vi "PIV_Stats_Single_Fast.vi"(0 "Data Folder":path=path "T:/Ensight_Data/NACA0015/NACA0015_NM_B/Test_A", 1 "PIV Meas Plane":enum16{"XY", "YZ", "XZ"}(ring)=enum."XZ", 2 "Row number":i32=1, 5 "Output Directory":path=path "T:/Ensight_Data/NACA0015/NACA0015_NM_B", 7 "XYZ Translation":dbl[](array[numeric])=[200.0, 8.0, -30.0], 9 "Case Name":string="Test_A_Case", 11 "PIV Freq (Hz)":dbl=7.25, 12 "Invert U":bool=TRUE, 13 "Invert V":bool) -> (4 "Progress Bar":i32(slide) scale=0.0..100.0, 6 "Status":string, 10 "# total vectors":i32=9858)   [LabVIEW 2022 SP3]
uses:
  <vilib>/Utility/error.llb/DialogType.ctl
  <vilib>/Analysis/1siggen.llb/Ramp Pattern by Samples.vi
  <vilib>/Utility/error.llb/Trim Whitespace One-Sided.vi
  <vilib>/Analysis/NI_AALBase.lvlib
panel:
  out "Data Array (spot,Var)":dbl[][](array[numeric])
  out "File Paths":path[](array[path])
  out "Position Array (XYZ,spot)":dbl[][](array[numeric])
  out "Variable Names":string[](array[string])=["Record_Length", "CHC", "u_ms", "v_ms", "time_s", "Vel_mag_ms", "Turb_Stats_U_ms", "Turb_Stats_u2_m2s2", "Turb_Stats_u3_m3s3", "Turb_Stats_u4_m4s4", "Turb_Stats_TurbU_%", "Turb_Stats_Skew_u", "Turb_Stats_Kurt_u", "Turb_Stats_V_ms", "Turb_Stats_v2_m2s2", "Turb_Stats_v3_m3s3", "Turb_Stats_v4_m4s4", "Turb_Stats_TurbV_%", "Turb_Stats_Skew_v", "Turb_Stats_Kurt_v", "Turb_Stats_u2v2_m4s4", "Turb_Stats_uv3_m4s4", "Turb_Stats_u3v_m4s4", "Turb_Stats_uv2_m3s3", "Turb_Stats_u2v_m3s3", "Turb_Stats_uv_cc", "Turb_Stats_uv", "Turb_Stats_TKE_J", "Turb_Stats_Error_U_ms", "Turb_Stats_Error_u2_m2s2", "Turb_Stats_Error_u3_m3s3", "Turb_Stats_Error_u4_m4s4", "Turb_Stats_Error_TurbU_%", "Turb_Stats_Error_Skew_u", "Turb_Stats_Error_Kurt_u", "Turb_Stats_Error_V_ms", "Turb_Stats_Error_v2_m2s2", "Turb_Stats_Error_v3_m3s3", "Turb_Stats_Error_v4_m4s4", "Turb_Stats_Error_TurbV_%", "Turb_Stats_Error_Skew_v", "Turb_Stats_Error_Kurt_v", "Turb_Stats_Error_u2v2_m4s4", "Turb_Stats_Error_uv3_m4s4", "Turb_Stats_Error_u3v_m4s4", "Turb_Stats_Error_uv2_m3s3", "Turb_Stats_Error_u2v_m3s3", "Turb_Stats_Error_uv_cc", "Turb_Stats_Error_uv", "Turb_Stats_Error_TKE_J"]
  out "time s":dbl[](array[numeric])=[0.0, 0.20689655172413793, 0.41379310344827586]
  out "File Array":path[](array[path])=[path "T:/Ensight_Data/NACA0015/NACA0015_NM_A/Test_A_Trans/New folder/Test_A000000.T076.D000.P000.H000.L.vec", path "T:/Ensight_Data/NACA0015/NACA0015_NM_A/Test_A_Trans/New folder/Test_A000001.T076.D000.P000.H000.L.vec", path "T:/Ensight_Data/NACA0015/NACA0015_NM_A/Test_A_Trans/New folder/Test_A000002.T076.D000.P000.H000.L.vec"]
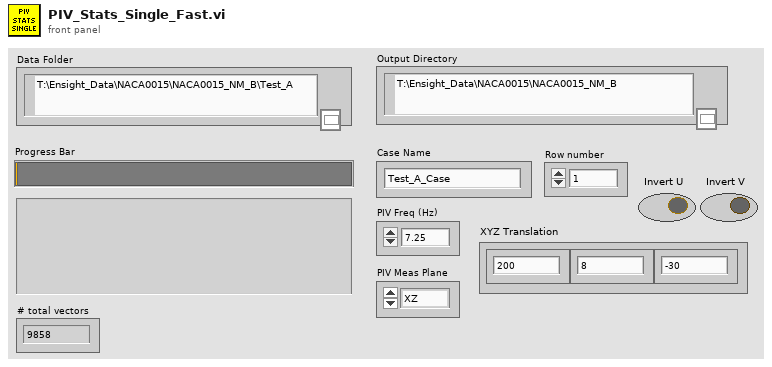
[diagram p1: front panel]
types:
  T1 = cluster{"Record Length":dbl, "CHC":dbl[], "u m/s":dbl[], "v m/s":dbl[], "time s":dbl[], "Vel mag m/s":dbl[], "XYZ Position":dbl[], " Turb Stats":cluster{"U m/s":dbl, "u2 m2/s2":dbl, "u3 m3/s3":dbl, "u4 m4/s4":dbl, "TurbU %":dbl, "Skew_u":dbl, "Kurt_u":dbl, "V m/s":dbl, "v2 m2/s2":dbl, "v3 m3/s3":dbl, "v4 m4/s4":dbl, "TurbV %":dbl, "Skew_v":dbl, "Kurt_v":dbl, "u2v2 m4/s4":dbl, "uv3 m4/s4":dbl, "u3v m4/s4":dbl, "uv2 m3/s3":dbl, "u2v m3/s3":dbl, "uv_cc":dbl, "uv":dbl, "TKE J":dbl}[], "Turb Stats Error":cluster{"U m/s":dbl, "u2 m2/s2":dbl, "u3 m3/s3":dbl, "u4 m4/s4":dbl, "TurbU %":dbl, "Skew_u":dbl, "Kurt_u":dbl, "V m/s":dbl, "v2 m2/s2":dbl, "v3 m3/s3":dbl, "v4 m4/s4":dbl, "TurbV %":dbl, "Skew_v":dbl, "Kurt_v":dbl, "u2v2 m4/s4":dbl, "uv3 m4/s4":dbl, "u3v m4/s4":dbl, "uv2 m3/s3":dbl, "u2v m3/s3":dbl, "uv_cc":dbl, "uv":dbl, "TKE J":dbl}[], "u (good)":dbl[], "v (good)":dbl[]}
  T2 = cluster{"Record Length":dbl, "CHC":dbl[], "u m/s":dbl[], "v m/s":dbl[], "time s":dbl[], "Vel mag m/s":dbl[], "XYZ Position":dbl[], " Turb Stats":cluster{"U m/s":dbl, "u2 m2/s2":dbl, "u3 m3/s3":dbl, "u4 m4/s4":dbl, "TurbU %":dbl, "Skew_u":dbl, "Kurt_u":dbl, "V m/s":dbl, "v2 m2/s2":dbl, "v3 m3/s3":dbl, "v4 m4/s4":dbl, "TurbV %":dbl, "Skew_v":dbl, "Kurt_v":dbl, "u2v2 m4/s4":dbl, "uv3 m4/s4":dbl, "u3v m4/s4":dbl, "uv2 m3/s3":dbl, "u2v m3/s3":dbl, "uv_cc":dbl, "uv":dbl, "TKE J":dbl}[], "Turb Stats Error":cluster{"U m/s":dbl, "u2 m2/s2":dbl, "u3 m3/s3":dbl, "u4 m4/s4":dbl, "TurbU %":dbl, "Skew_u":dbl, "Kurt_u":dbl, "V m/s":dbl, "v2 m2/s2":dbl, "v3 m3/s3":dbl, "v4 m4/s4":dbl, "TurbV %":dbl, "Skew_v":dbl, "Kurt_v":dbl, "u2v2 m4/s4":dbl, "uv3 m4/s4":dbl, "u3v m4/s4":dbl, "uv2 m3/s3":dbl, "u2v m3/s3":dbl, "uv_cc":dbl, "uv":dbl, "TKE J":dbl}[], "u (good)":dbl[], "v (good)":dbl[]}[]
  T3 = cluster{"U m/s":dbl, "u2 m2/s2":dbl, "u3 m3/s3":dbl, "u4 m4/s4":dbl, "TurbU %":dbl, "Skew_u":dbl, "Kurt_u":dbl, "V m/s":dbl, "v2 m2/s2":dbl, "v3 m3/s3":dbl, "v4 m4/s4":dbl, "TurbV %":dbl, "Skew_v":dbl, "Kurt_v":dbl, "u2v2 m4/s4":dbl, "uv3 m4/s4":dbl, "u3v m4/s4":dbl, "uv2 m3/s3":dbl, "u2v m3/s3":dbl, "uv_cc":dbl, "uv":dbl, "TKE J":dbl}
  T4 = cluster{"U m/s":dbl, "u2 m2/s2":dbl, "u3 m3/s3":dbl, "u4 m4/s4":dbl, "TurbU %":dbl, "Skew_u":dbl, "Kurt_u":dbl, "V m/s":dbl, "v2 m2/s2":dbl, "v3 m3/s3":dbl, "v4 m4/s4":dbl, "TurbV %":dbl, "Skew_v":dbl, "Kurt_v":dbl, "u2v2 m4/s4":dbl, "uv3 m4/s4":dbl, "u3v m4/s4":dbl, "uv2 m3/s3":dbl, "u2v m3/s3":dbl, "uv_cc":dbl, "uv":dbl, "TKE J":dbl}[]
  T5 = typedef "DialogType.ctl" = u16
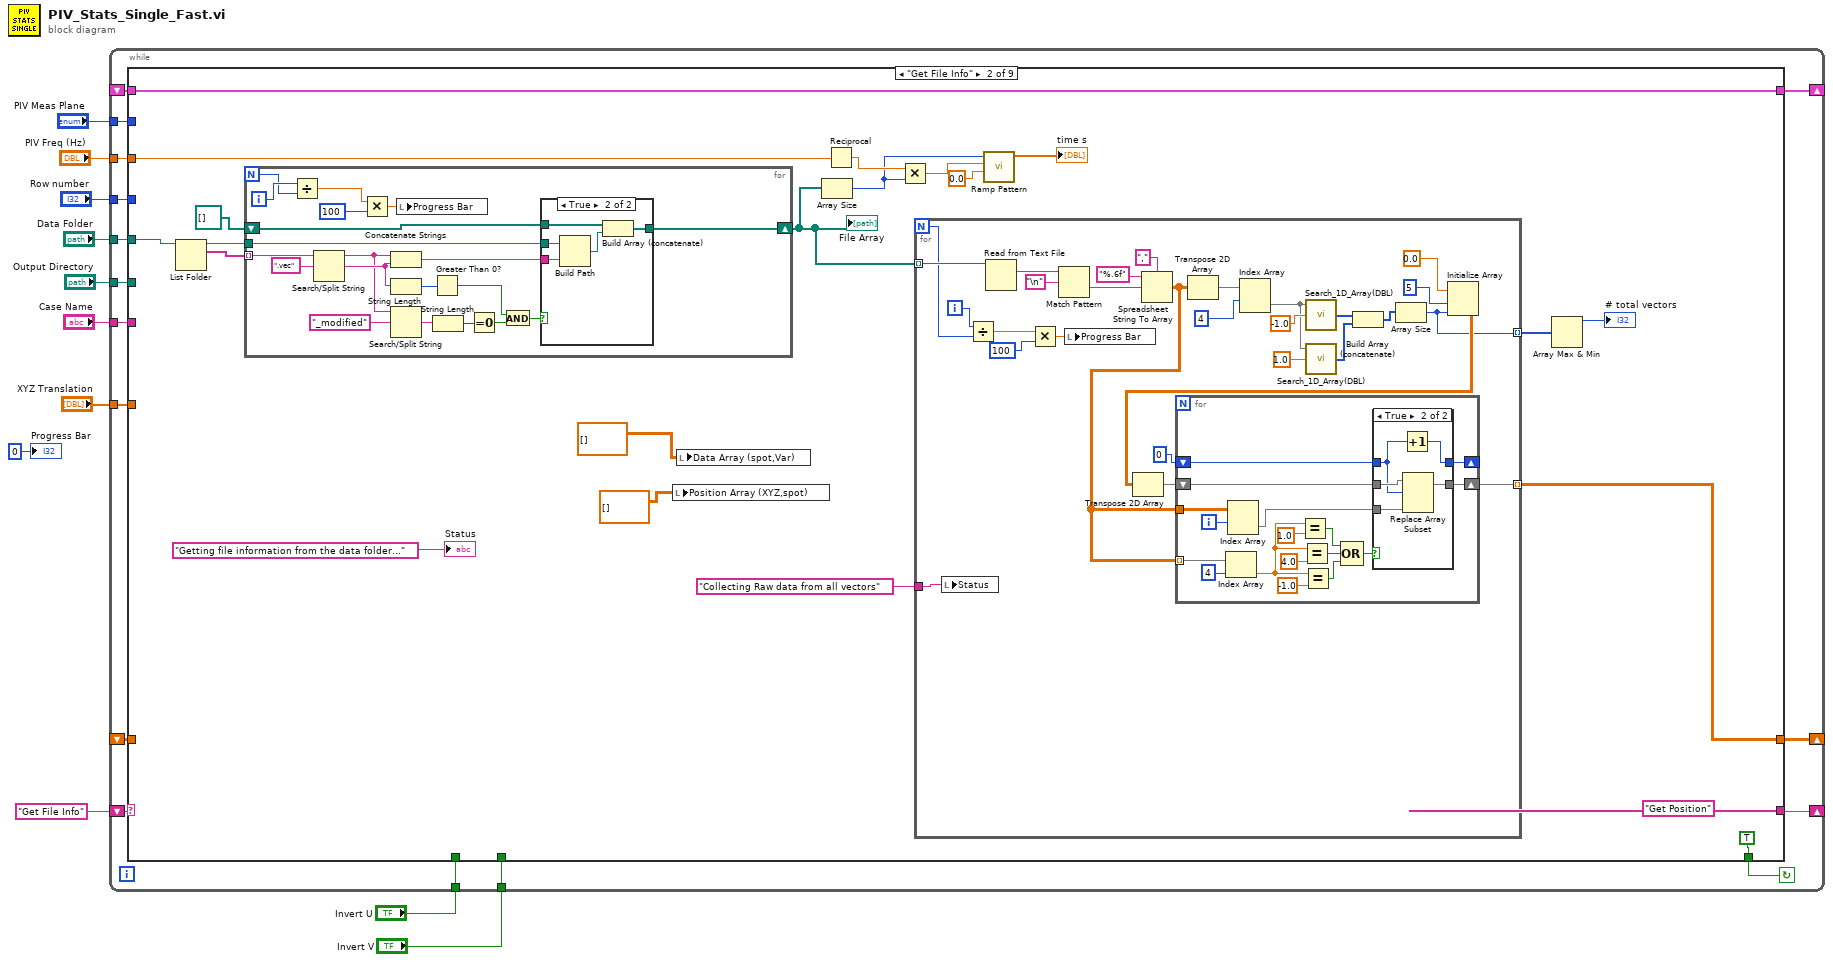
[diagram p0: block diagram]
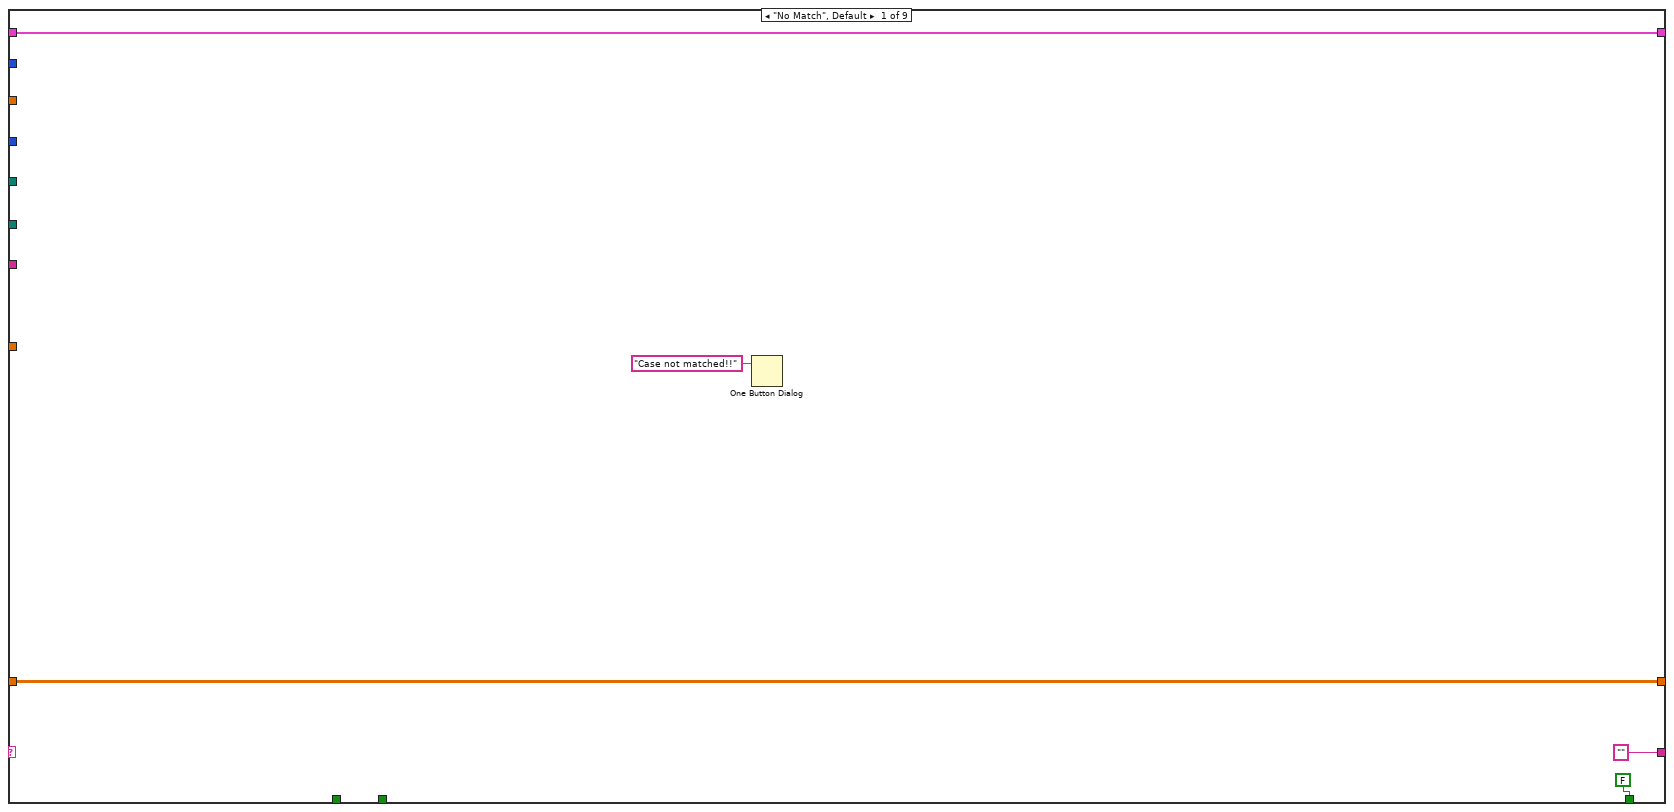
[diagram p2: hidden frame]
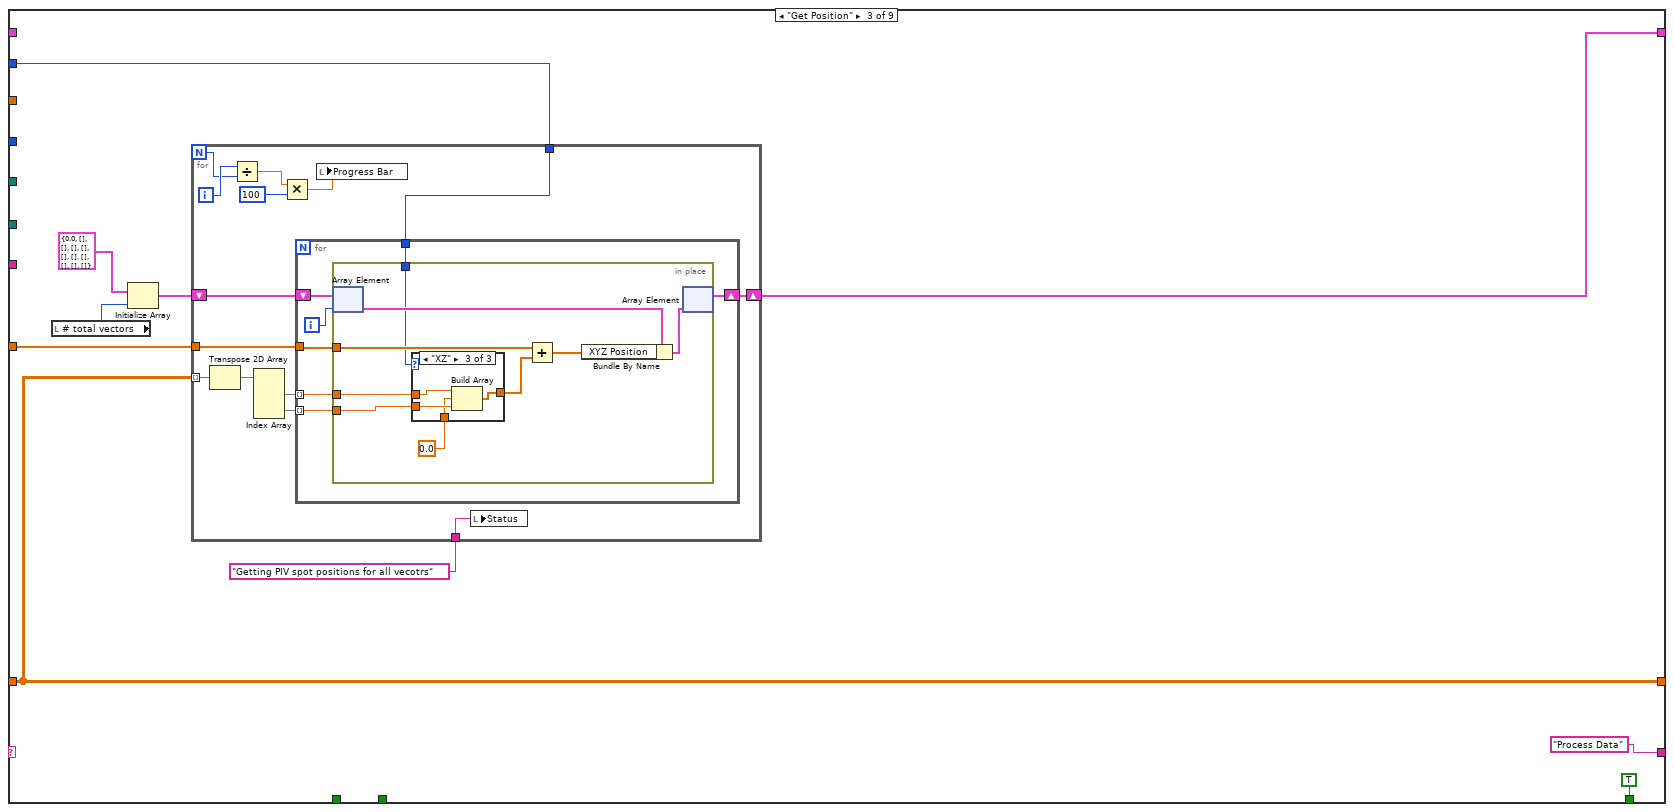
[diagram p5: hidden frame]
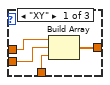
[diagram p6: hidden frame]
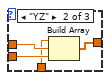
[diagram p7: hidden frame]
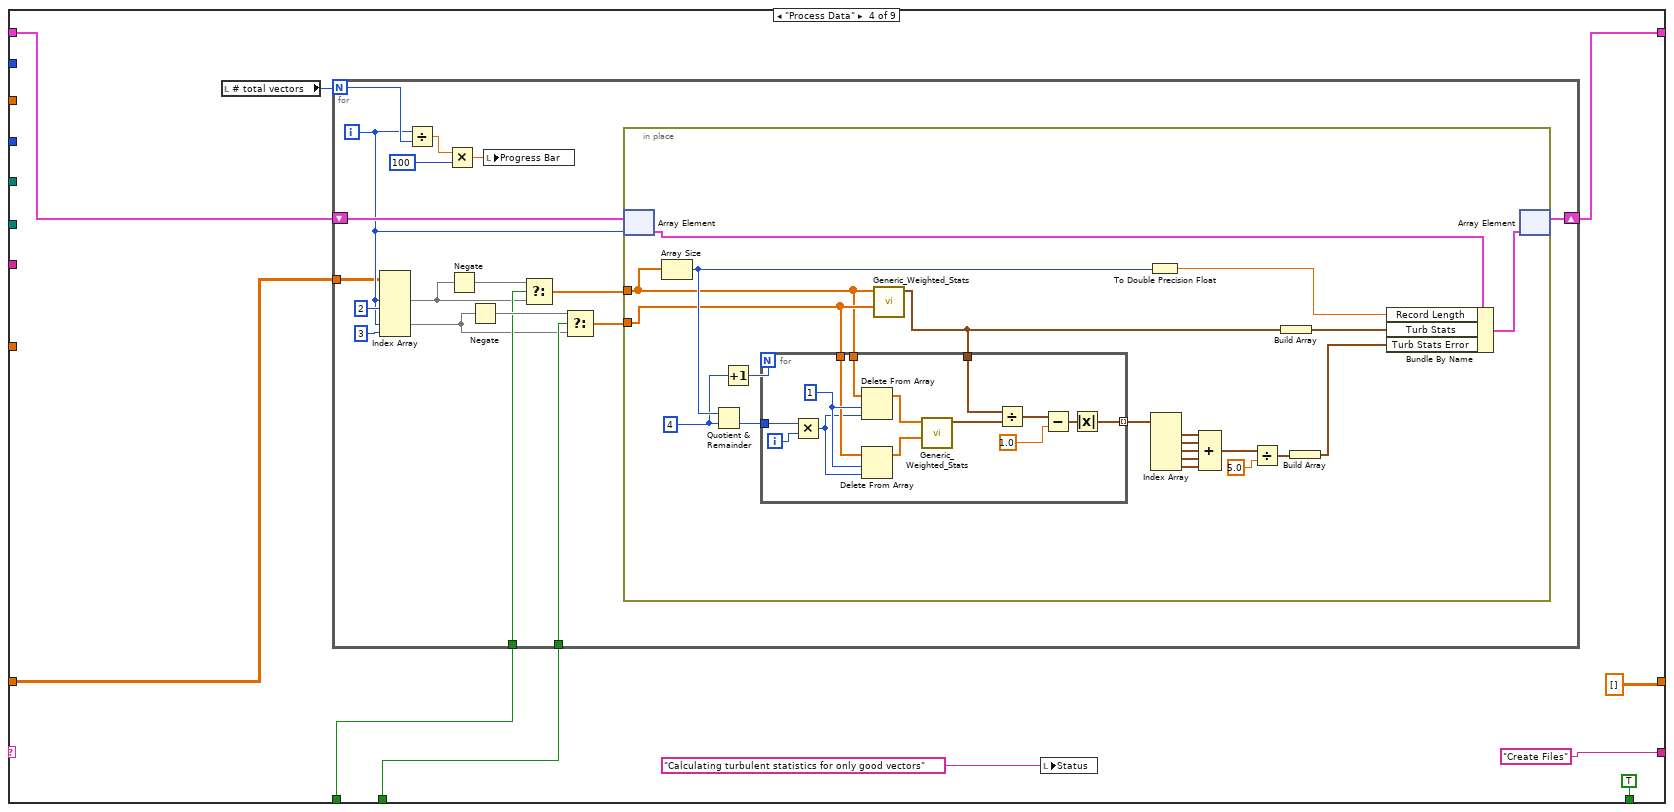
[diagram p8: hidden frame]
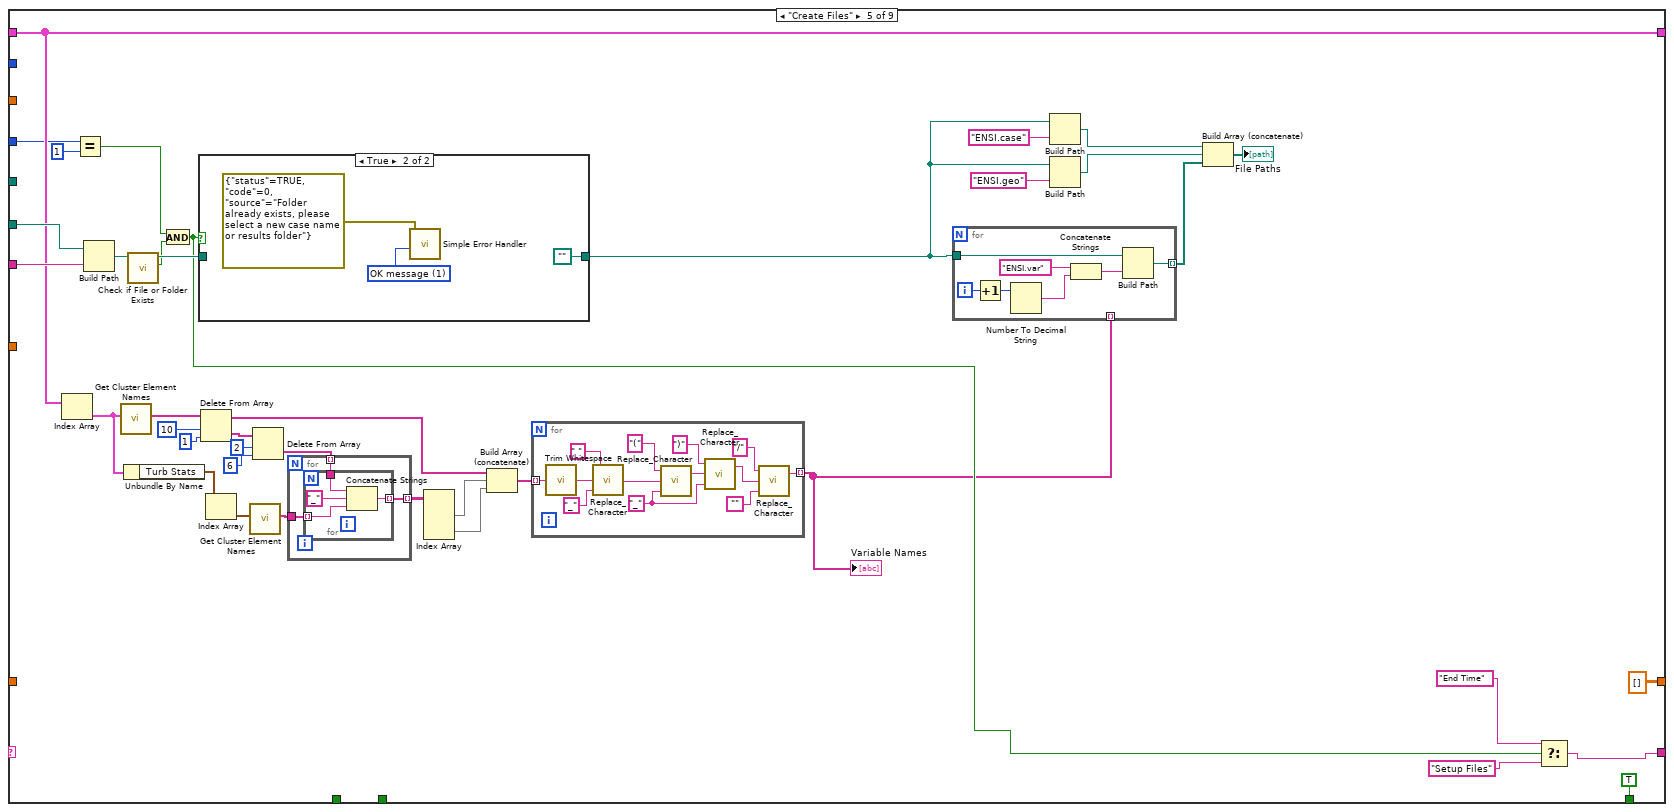
[diagram p9: hidden frame]
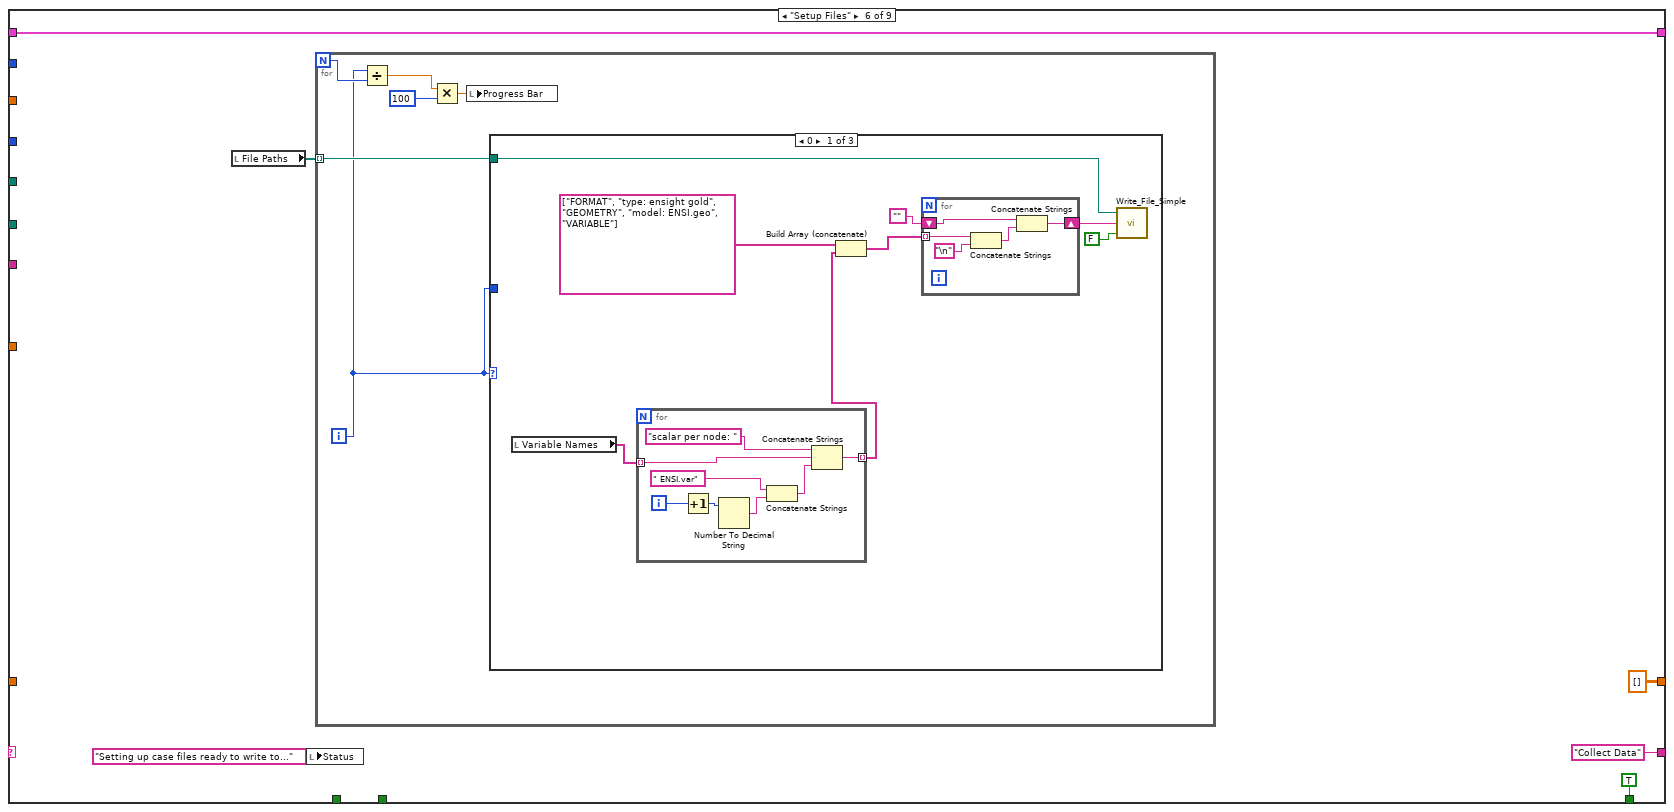
[diagram p11: hidden frame]
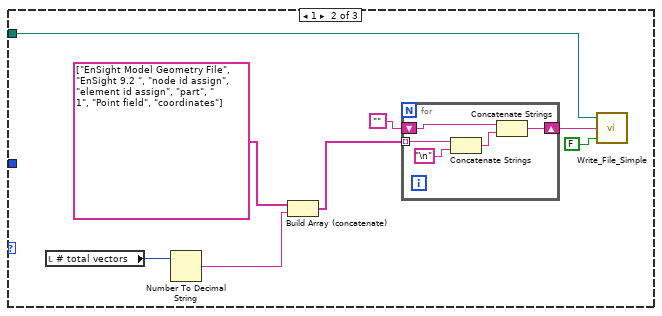
[diagram p12: hidden frame]
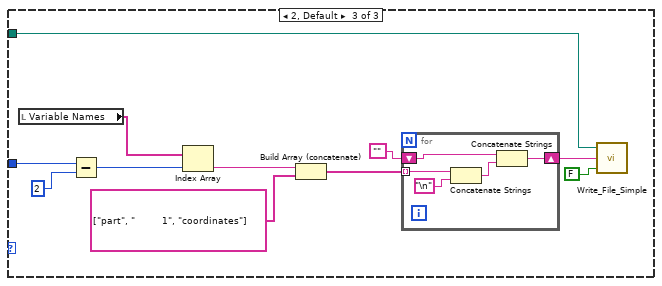
[diagram p13: hidden frame]
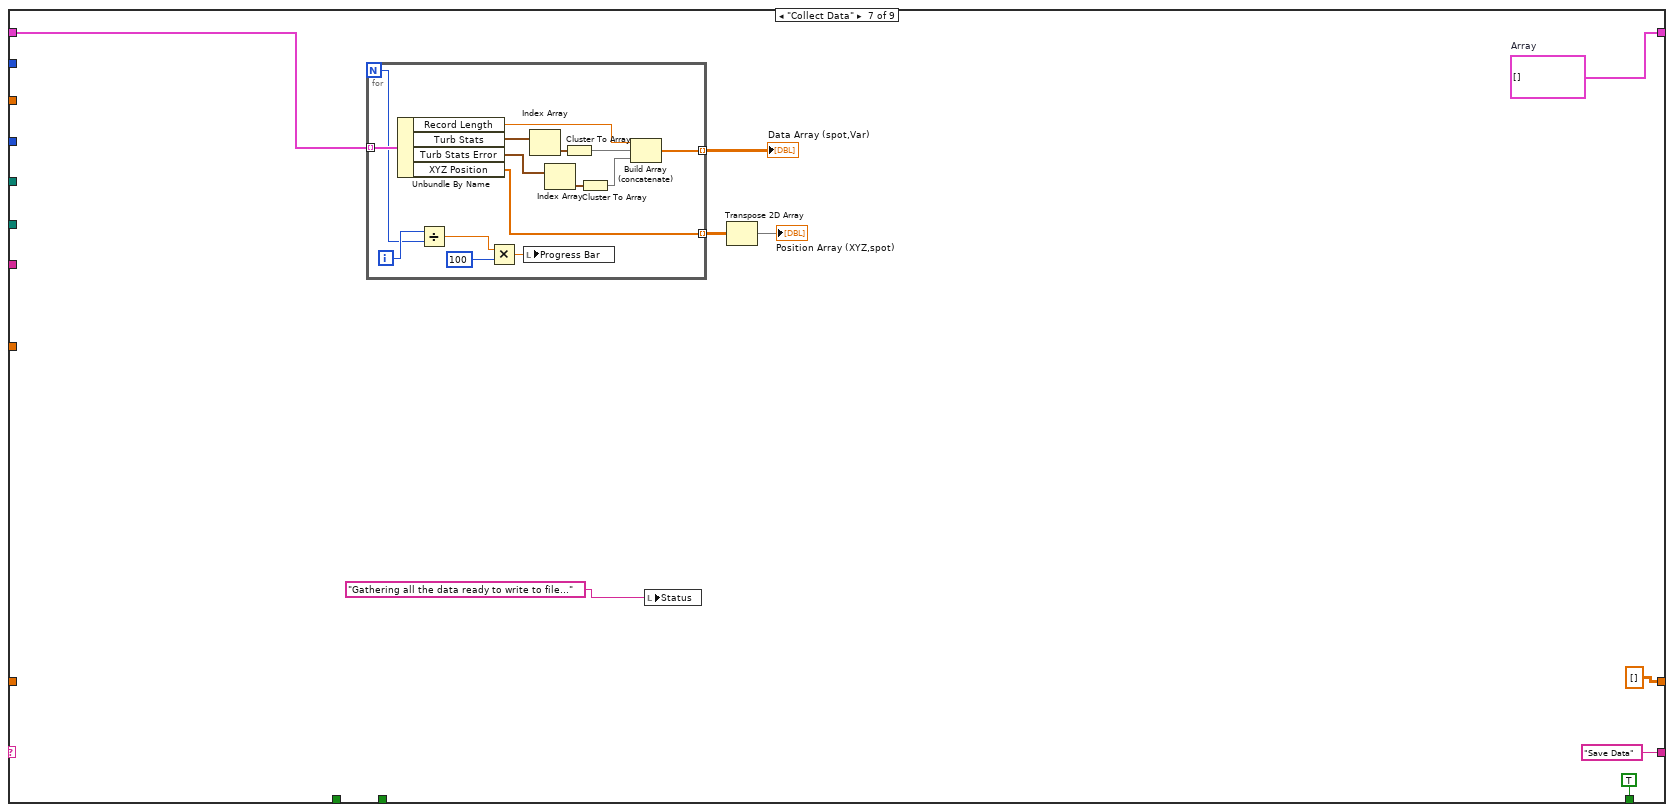
[diagram p14: hidden frame]
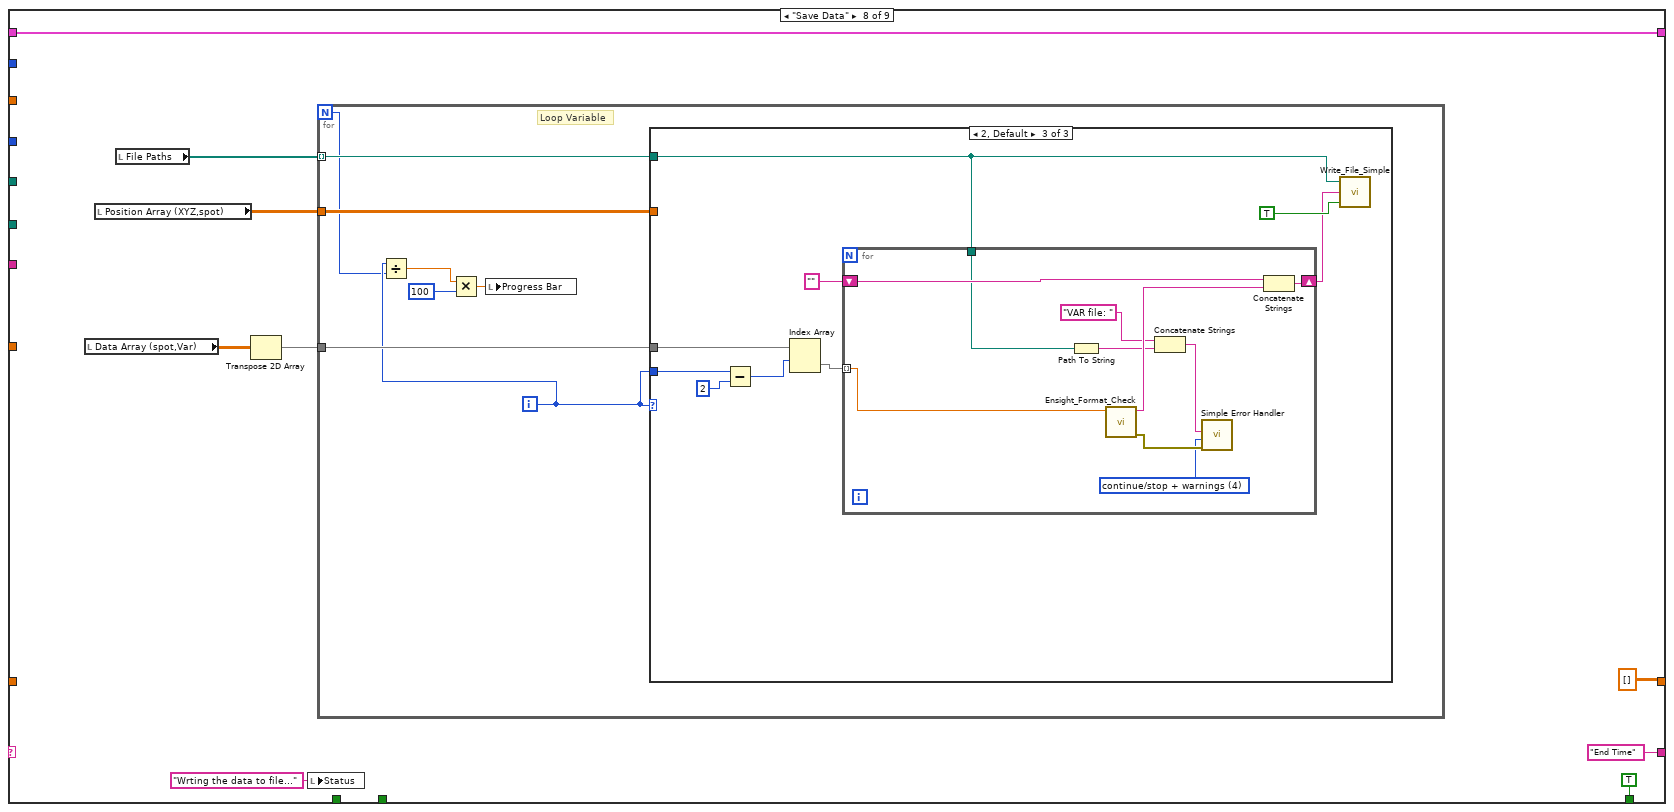
[diagram p15: hidden frame]
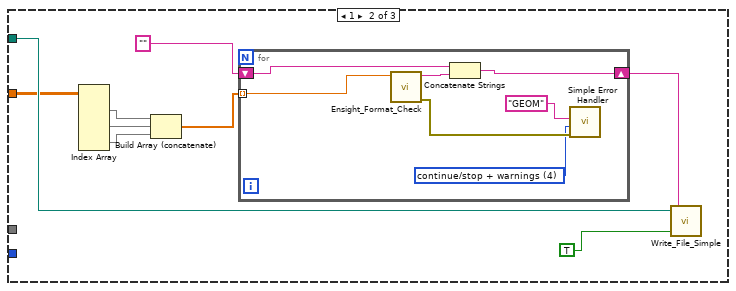
[diagram p17: hidden frame]
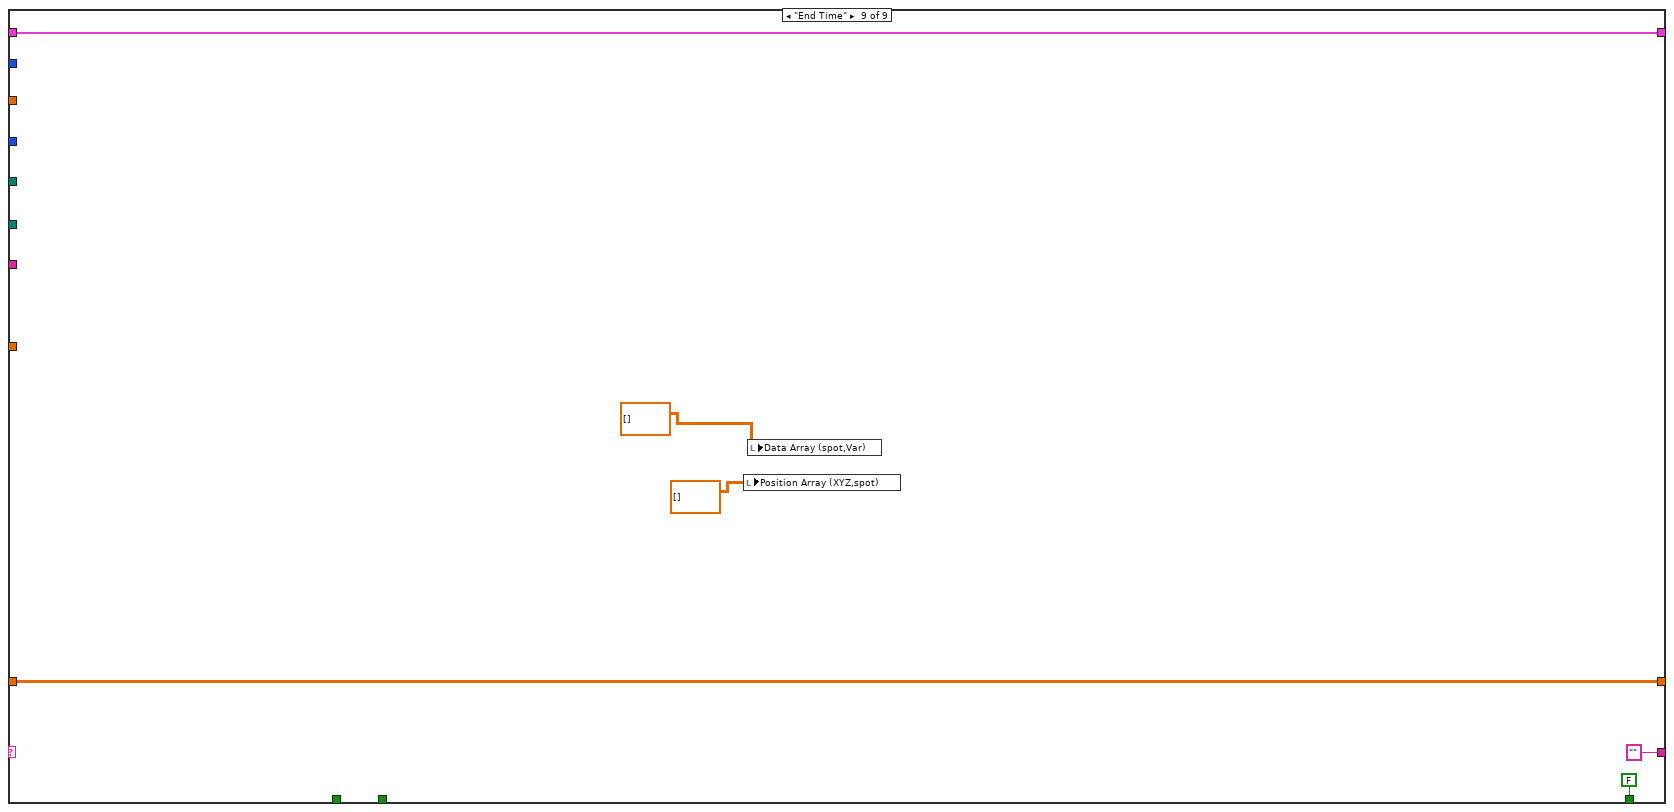
[diagram p18: hidden frame]
diagram:
  n1 = while {
    shift-right: [w26] -> _
    shift-left: "Get File Info" -> [w27]
    tunnel: "Data Folder" -> [w25]
    tunnel: "Output Directory" -> [w23]
    tunnel: "Case Name" -> [w22]
    tunnel: "PIV Freq (Hz)" -> [w21]
    tunnel: "PIV Meas Plane" -> [w20]
    tunnel: "XYZ Translation" -> [w19]
    shift-right: [w18] -> _
    shift-left: _ -> [w17]
    tunnel: "Row number" -> [w16]
    tunnel: "Invert V" -> [w15]
    tunnel: "Invert U" -> [w14]
    shift-right: [w13] -> _
    shift-left: _ -> [w12]
    stop <- w24 continue-if-true
    n2 = case shown="\"Get File Info\"" w27 {
      tunnel: ["" "Get Position" "Process Data" "Create Files" w260 "Collect Data" ("t") "Save Data" ("t") "End Time" ("t") "" ("t")] -> w26
      tunnel: w25 -> [_ w48 _ _ _ _ _ _ _]
      tunnel: [FALSE TRUE TRUE TRUE TRUE TRUE TRUE TRUE FALSE] -> w24
      tunnel: w23 -> [_ _ _ _ w284 _ _ _ _]
      tunnel: w22 -> [_ _ _ _ w285 _ _ _ _]
      tunnel: w21 -> [_ w47 _ _ _ _ _ _ _]
      tunnel: w20 -> [_ _ w138 _ _ _ _ _ _]
      tunnel: w19 -> [_ _ w139 _ _ _ _ _ _]
      tunnel: [w30 w35 w133 w192 w270 w319 w383 w409 w456] -> w18
      tunnel: w17 -> [w30 w35 _ w190 w270 w319 w385 w409 w456]
      tunnel: w16 -> [_ _ _ _ w266 _ _ _ _]
      tunnel: w15 -> [_ _ _ w189 _ _ _ _ _]
      tunnel: w14 -> [_ _ _ w188 _ _ _ _ _]
      tunnel: [w28 w33 w132 dbl[][][] [] ("GoodRawData(time,spot)") dbl[][][] [] ("GoodRawData(time,spot)") dbl[][][] [] ("GoodRawData(time,spot)") dbl[][][] [] ("GoodRawData(time,spot)") dbl[][][] [] ("GoodRawData(time,spot)") w455] -> w13
      tunnel: w12 -> [w28 _ w132 w185 _ _ _ _ w455]
      frame "No Match", Default {
        n3 = One Button Dialog(message="Case not matched!!") -> ()  [unwired: 1 in, 1 out]
      }
      frame "Get File Info" {
        n4 = List Folder(path=w48) -> (path out=w50:path, filenames=w51:string[])  [unwired: 3 in, 2 out]
        n5 = for {
          N -> [w106]
          tunnel: w51 -> [w125] mode=indexing
          shift-right: [w118] -> w38
          shift-left: path[] [] -> [w120]
          tunnel: w50 -> [w119]
          i -> [w107]
          n6 = Divide(x=w107, y=w106) -> (x/y=w109:dbl)
          n7 = Search/Split String(string=w125, search string/char (-)=".vec") -> (substring before match=w116:string, match + rest of string=w122:string)  [unwired: 1 in, 1 out]
          n8 = Multiply(x=w109, y=100) -> (x*y=w110:dbl)
          n9 = Concatenate Strings(w116, w122) -> (w121:string)
          n10 = String Length(string=w122) -> (length=w123:i32)
          n11 = Search/Split String(string=w116, search string/char (-)="_modified") -> (match + rest of string=w114:string)  [unwired: 1 in, 2 out]
          n12 = local write "Progress Bar"(w110) -> ()
          n13 = Greater Than 0?(x=w123) -> (x > 0?=w117:bool)
          n14 = String Length(string=w114) -> (length=w113:i32)
          n15 = Equal To 0?(x=w113) -> (x = 0?=w112:bool)
          n16 = And(x=w117, y=w112) -> (x .and. y?=w111:bool)
          n17 = case shown="True" w111 {
            tunnel: w121 -> [_ w131]
            tunnel: w120 -> [w126 w127]
            tunnel: w119 -> [_ w130]
            tunnel: [w126 w128] -> w118
            frame False {
            }
            frame True {
              n18 = Build Path(base path=w130, name or relative path=w131) -> (appended path=w129:path)
              n19 = Build Array (concatenate)(w127, w129) -> (w128:path[])
            }
          }
        }
        "File Array" <- w38
        n20 = local write "Position Array (XYZ,spot)"(dbl[][] [] ("Position Array")) -> ()
        n21 = local write "Data Array (spot,Var)"(dbl[][] [] ("Data Array")) -> ()
        n22 = Array Size(array=w38) -> (size(s)=w42:i32)
        n23 = Reciprocal(x=w47) -> (1/x=w45:dbl)
        n24 = Multiply(x=w45, y=w42) -> (x*y=w46:dbl)
        n25 = for {
          N -> [w65]
          tunnel: w38 -> [w72] mode=indexing
          tunnel: [w54] -> w37 mode=indexing
          tunnel: [w69] -> w33 mode=indexing
          tunnel: "Collecting Raw data from all vectors" ("Status") -> [w63]
          i -> [w64]
          n26 = local write "Status"(w63) -> ()
          n27 = Divide(x=w64, y=w65) -> (x/y=w67:dbl)
          n28 = Read from Text File(file (use dialog)=w72) -> (text=w81:string)  [unwired: 3 in, 3 out]
          n29 = Multiply(x=w67, y=100) -> (x*y=w66:dbl)
          n30 = Match Pattern(string=w81, regular expression="\n") -> (after substring=w77:string)  [unwired: 1 in, 3 out]
          n31 = local write "Progress Bar"(w66) -> ()
          n32 = Spreadsheet String To Array(delimiter (Tab)=",", format string="%.6f", spreadsheet string=w77) -> (array=w60:dbl[][])  [unwired: 1 in]
          n33 = Transpose 2D Array(2D array=w60) -> (transposed array=w76:dbl[][])
          n34 = Index Array(array=w76, index (row)=4) -> (element=w59:dbl[])  [unwired: 1 in]
          n35 = call "Search_1D_Array(DBL).vi"("Array"=w59, "Element Data"=-1.0) -> ("Indicies of Elements"=w58:i32[])  [unwired: 6 in, 1 out]
          n36 = call "Search_1D_Array(DBL).vi"("Array"=w59, "Element Data"=1.0) -> ("Indicies of Elements"=w56:i32[])  [unwired: 6 in, 1 out]
          n37 = Build Array (concatenate)(w58, w56) -> (w57:i32[])
          n38 = Array Size(array=w57) -> (size(s)=w54:i32)
          n39 = Initialize Array(0.0 ("element"), 5 ("dimension size"), w54) -> (w70:dbl[][])
          n40 = Transpose 2D Array(2D array=w70) -> (transposed array=w71:dbl[][])
          n41 = for {
            tunnel: w60 -> [w93] mode=indexing
            shift-right: [w96] -> w69
            shift-left: w71 -> [w91]
            shift-right: [w95] -> _
            shift-left: 0 ("y") -> [w94]
            tunnel: w60 -> [w92]
            i -> [w90]
            n42 = Index Array(array=w93, index=4) -> (element=w87:dbl)
            n43 = Index Array(array=w92, index (row)=w90) -> (element=w97:dbl[])  [unwired: 1 in]
            n44 = Equal?(x=w87, y=1.0) -> (x = y?=w83:bool)
            n45 = Equal?(x=w87, y=4.0) -> (x = y?=w84:bool)
            n46 = Equal?(x=w87, y=-1.0) -> (x = y?=w85:bool)
            n47 = Compound Arithmetic op=OR(w83, w84, w85) -> (w82:bool)
            n48 = case shown="True" w82 {
              tunnel: w97 -> [_ w103]
              tunnel: w91 -> [w100 w105]
              tunnel: [w100 w104] -> w96
              tunnel: [w99 w102] -> w95
              tunnel: w94 -> [w99 w101]
              frame False {
              }
              frame True {
                n49 = Increment(x=w101) -> (x+1=w102:i32)
                n50 = Replace Array Subset(array=w105, new element=w103, index (row)=w101) -> (w104:dbl[][])  [unwired: 1 in]
              }
            }
          }
        }
        n51 = call-poly <vilib>:"Ramp Pattern.vi"("start"=0.0, "end"=w46, "samples"=w42) -> ("Ramp Pattern"=→"time s":dbl[])  [unwired: 7 in, 1 out]
        n52 = Array Max & Min(array=w37) -> (max value=→"# total vectors":i32)  [unwired: 3 out]
        "Status" <- "Getting file information from the data folder..." ("Status")
      }
      frame "Get Position" {
        n53 = local read "# total vectors"() -> (w137:i32)
        n54 = Initialize Array(T1 {"Record Length"=0.0, "CHC"=[], "u m/s"=[], "v m/s"=[], "time s"=[], "Vel mag m/s"=[], "XYZ Position"=[], " Turb Stats"=[], "Turb Stats Error"=[], "u (good)"=[], "v (good)"=[]} ("Spot Data Cluster"), w137) -> (w135:T2)
        n55 = for {
          N -> [w146]
          shift-right: [w151] -> w133
          shift-left: w135 -> [w152]
          tunnel: w132 -> [w144] mode=indexing
          tunnel: w139 -> [w153]
          tunnel: w138 -> [w145]
          tunnel: "Getting PIV spot positions for all vecotrs" ("Status") -> [w142]
          i -> [w147]
          n56 = Transpose 2D Array(2D array=w144) -> (transposed array=w143:dbl[][])
          n57 = Divide(x=w147, y=w146) -> (x/y=w149:dbl)
          n58 = Index Array(array=w143) -> (element #1=w155:dbl[], element #2=w154:dbl[])  [unwired: 4 in]
          n59 = Multiply(x=w149, y=100) -> (x*y=w150:dbl)
          n60 = for {
            tunnel: w155 -> [w162] mode=indexing
            tunnel: w154 -> [w161] mode=indexing
            tunnel: w153 -> [w160]
            shift-right: [w157] -> w151
            shift-left: w152 -> [w159]
            tunnel: w145 -> [w156]
            i -> [w158]
            n61 = in-place {
              in-place-border: w162 -> [w169]
              in-place-border: w161 -> [w168]
              in-place-border: w160 -> [w167]
              in-place-border: w156 -> [w163]
              n62 = in-place-array #1(w159, w158) -> (w166:T1)
              n63 = case shown="\"XZ\"" w163 {
                tunnel: w169 -> [w173 w179 w183]
                tunnel: w168 -> [w174 w178 w182]
                tunnel: 0.0 ("element") -> [w175 w177 w181]
                tunnel: [w172 w176 w180] -> w171
                frame "XY" {
                  n64 = Build Array(w173, w174, w175) -> (w172:dbl[])
                }
                frame "YZ" {
                  n65 = Build Array(w177, w179, w178) -> (w176:dbl[])
                }
                frame "XZ" {
                  n66 = Build Array(w183, w181, w182) -> (w180:dbl[])
                }
              }
              n67 = Add(x=w167, y=w171) -> (x+y=w165:dbl[])
              n68 = Bundle By Name(cluster=w166, "XYZ Position"=w165) -> (w164:T1)
              n69 = in-place-array #1(w164) -> (w157:T2)  [unwired: 1 out]
            }
          }
          n70 = local write "Progress Bar"(w150) -> ()
          n71 = local write "Status"(w142) -> ()
        }
      }
      frame "Process Data" {
        n72 = local read "# total vectors"() -> (w184:i32)
        n73 = for {
          N: w184 -> [w202]
          tunnel: w189 -> [w201]
          tunnel: w188 -> [w200]
          tunnel: w185 -> [w194]
          shift-right: [w206] -> w192
          shift-left: w190 -> [w211]
          i -> [w195]
          n74 = Index Array(array=w194, index (dim 1) #1=w195, index (dim 2) #1=2 ("disabled index (col)"), index (dim 1) #2=w195, index (dim 2) #2=3 ("disabled index (col)")) -> (element #1=w197:dbl[], element #2=w196:dbl[])  [unwired: 2 in]
          n75 = Divide(x=w195, y=w202) -> (x/y=w204:dbl)
          n76 = Multiply(x=w204, y=100) -> (x*y=w205:dbl)
          n77 = Negate(x=w197) -> (-x=w210:dbl[])
          n78 = Negate(x=w196) -> (-x=w209:dbl[])
          n79 = local write "Progress Bar"(w205) -> ()
          n80 = Select(t=w210, s=w200, f=w197) -> (s? t:f=w208:dbl[])
          n81 = Select(t=w209, s=w201, f=w196) -> (s? t:f=w207:dbl[])
          n82 = in-place {
            in-place-border: w208 -> [w225]
            in-place-border: w207 -> [w226]
            w227 = 4 ("y")
            n83 = in-place-array #2(w211, w195) -> (w232:T1)
            n84 = Array Size(array=w225) -> (size(s)=w229:i32)
            n85 = Quotient & Remainder(x=w229, y=w227) -> (floor(x/y)=w223:i32)  [unwired: 1 out]
            n86 = Increment(x=w227) -> (x+1=w228:i32)
            n87 = call "Generic_Weighted_Stats.vi"("v"=w226, "u"=w225) -> ("Turbulence Statistics"=w222:T3)  [unwired: 9 in]
            n88 = for {
              N: w228 -> [_]
              tunnel: w222 -> [w241]
              tunnel: w223 -> [w239]
              tunnel: w225 -> [w236]
              tunnel: w226 -> [w235]
              tunnel: [w233] -> w221 mode=indexing
              i -> [w238]
              w237 = 1 ("y")
              n89 = Multiply(x=w239, y=w238) -> (x*y=w234:i32)
              n90 = Delete From Array(array=w236, length=w237, index=w234) -> (array with subset deleted=w246:dbl[])  [unwired: 1 out]
              n91 = Delete From Array(array=w235, length=w237, index=w234) -> (array with subset deleted=w245:dbl[])  [unwired: 1 out]
              n92 = call "Generic_Weighted_Stats.vi"("v"=w245, "u"=w246) -> ("Turbulence Statistics"=w240:T3)  [unwired: 9 in]
              n93 = Divide(x=w241, y=w240) -> (x/y=w242:T3)
              n94 = Subtract(x=w242, y=1.0 ("Record Length")) -> (x-y=w244:T3)
              n95 = Absolute Value(x=w244) -> (abs(x)=w233:T3)
            }
            n96 = To Double Precision Float(number=w229) -> (double precision float=w230:dbl)
            n97 = Index Array(array=w221) -> (element #1=w220:T3, element #2=w219:T3, element #3=w218:T3, element #4=w217:T3, element #5=w216:T3)  [unwired: 5 in]
            n98 = Compound Arithmetic op=ADD(w220, w219, w218, w217, w216) -> (w215:T3)
            n99 = Divide(x=w215, y=5.0 ("Record Length")) -> (x/y=w213:T3)
            n100 = Build Array(w222) -> (w224:T4)
            n101 = Build Array(w213) -> (w212:T4)
            n102 = Bundle By Name(cluster=w232, "Record Length"=w230, "Turb Stats"=w224, "Turb Stats Error"=w212) -> (w231:T1)
            n103 = in-place-array #2(w231) -> (w206:T2)  [unwired: 1 out]
          }
        }
        n104 = local write "Status"("Calculating turbulent statistics for only good vectors" ("Status")) -> ()
      }
      frame "Create Files" {
        n105 = Index Array(array=w270) -> (element=w282:T1)  [unwired: 1 in]
        n106 = Equal?(x=w266, y=1) -> (x = y?=w261:bool)
        n107 = Build Path(base path=w284, name or relative path=w285) -> (appended path=w264:path)
        n108 = call "Get Cluster Element Names.vi"("Cluster"=w282) -> ("Element Names"=w281:string[])  [unwired: 9 in, 1 out]
        n109 = Unbundle By Name(w282) -> ("Turb Stats"=w272:T4)
        n110 = call <vilib>:"Check if File or Folder Exists.vi"("path"=w264) -> ("file or folder exists?"=w262:bool, "dup path"=w263:path)  [unwired: 8 in, 1 out]
        n111 = And(x=w261, y=w262) -> (x .and. y?=w258:bool)
        n112 = case shown="True" w258 {
          tunnel: [w293 path "" ("dup path")] -> w250
          tunnel: w263 -> [w293 _]
          frame False {
          }
          frame True {
            w296 = T5 1 items=["no dialog", "OK message", "continue or stop message", "OK message + warnings", "continue/stop + warnings"] ("type of dialog (OK msg:1)")
            n113 = call <vilib>:"Simple Error Handler.vi"("type of dialog (OK msg:1)"=w296, "error in (no error)"=errorcluster {"status"=TRUE, "code"=0, "source"="Folder already exists, please select a new case name or results folder"}) -> ()  [unwired: 3 in, 5 out]
          }
        }
        n114 = Delete From Array(array=w281, length=10, index=1) -> (deleted portion=w269:string[], array with subset deleted=w277:string[])
        n115 = Index Array(array=w272) -> (element=w271:T3)  [unwired: 1 in]
        n116 = call "Get Cluster Element Names.vi"("Cluster"=w271) -> ("Element Names"=w278:string[])  [unwired: 9 in, 1 out]
        n117 = Delete From Array(array=w269, length=2, index=6) -> (deleted portion=w247:string[])  [unwired: 1 out]
        n118 = for {
          tunnel: w247 -> [w299] mode=indexing
          tunnel: w278 -> [w298]
          tunnel: [w297] -> w276 mode=indexing
          n119 = for {
            tunnel: w299 -> [w303]
            tunnel: w298 -> [w301] mode=indexing
            tunnel: [w300] -> w297 mode=indexing
            n120 = Concatenate Strings(w303, "_" ("string"), w301) -> (w300:string)
          }
        }
        n121 = Index Array(array=w276) -> (element #1=w275:string[], element #2=w274:string[])  [unwired: 4 in]
        n122 = Build Array (concatenate)(w277, w275, w274) -> (w273:string[])
        n123 = for {
          tunnel: w273 -> [w306] mode=indexing
          tunnel: [w308] -> w251 mode=indexing
          w312 = "_" ("Replace with")
          n124 = call <vilib>:"Trim Whitespace.vi"("string"=w306) -> ("trimmed string"=w304:string)  [unwired: 1 in]
          n125 = call "Replace_Character.vi"("Replace with"="_", "Input String"=w304, "Search For"=" ") -> ("Output string"=w307:string)  [unwired: 1 out]
          n126 = call "Replace_Character.vi"("Replace with"=w312, "Input String"=w307, "Search For"="(") -> ("Output string"=w314:string)  [unwired: 1 out]
          n127 = call "Replace_Character.vi"("Replace with"=w312, "Input String"=w314, "Search For"=")") -> ("Output string"=w311:string)  [unwired: 1 out]
          n128 = call "Replace_Character.vi"("Replace with"="", "Input String"=w311, "Search For"="/") -> ("Output string"=w308:string)  [unwired: 1 out]
        }
        "Variable Names" <- w251
        n129 = for {
          tunnel: w250 -> [w292]
          tunnel: [w286] -> w256 mode=indexing
          tunnel: w251 -> [_] mode=indexing
          i -> [w291]
          n130 = Increment(x=w291) -> (x+1=w290:i32)
          n131 = Number To Decimal String(number=w290) -> (decimal integer string=w288:string)  [unwired: 1 in]
          n132 = Concatenate Strings("ENSI.var" ("name or relative path"), w288) -> (w287:string)
          n133 = Build Path(base path=w292, name or relative path=w287) -> (appended path=w286:path)
        }
        n134 = Build Path(base path=w250, name or relative path="ENSI.case") -> (appended path=w254:path)
        n135 = Build Path(base path=w250, name or relative path="ENSI.geo") -> (appended path=w255:path)
        n136 = Build Array (concatenate)(w254, w255, w256) -> (→"File Paths":path[])
        n137 = Select(t="End Time", s=w258, f="Setup Files" ("t")) -> (s? t:f=w260:string)
      }
      frame "Setup Files" {
        n138 = local read "File Paths"() -> (w322:path[])
        n139 = local write "Status"("Setting up case files ready to write to..." ("Status")) -> ()
        n140 = for {
          N -> [w325]
          tunnel: w322 -> [w328] mode=indexing
          i -> [w323]
          n141 = Divide(x=w323, y=w325) -> (x/y=w324:dbl)
          n142 = Multiply(x=w324, y=100) -> (x*y=w327:dbl)
          n143 = local write "Progress Bar"(w327) -> ()
          n144 = case shown="0" w323 {
            tunnel: w328 -> [w333 w354 w373]
            tunnel: w323 -> [_ _ w368]
            frame 0 {
              n145 = local read "Variable Names"() -> (w330:string[])
              n146 = for {
                tunnel: w330 -> [w339] mode=indexing
                tunnel: [w337] -> w329 mode=indexing
                i -> [w342]
                n147 = Increment(x=w342) -> (x+1=w343:i32)
                n148 = Number To Decimal String(number=w343) -> (decimal integer string=w340:string)  [unwired: 1 in]
                n149 = Concatenate Strings(" ENSI.var", w340) -> (w338:string)
                n150 = Concatenate Strings("scalar per node: ", w339, w338) -> (w337:string)
              }
              n151 = Build Array (concatenate)(string[] ["FORMAT", "type: ensight gold", "GEOMETRY", "model: ENSI.geo", "VARIABLE"], w329) -> (w332:string[])
              n152 = for {
                tunnel: w332 -> [w349] mode=indexing
                shift-right: [w347] -> w335
                shift-left: "" -> [w345]
                n153 = Concatenate Strings(w349, "\n") -> (w346:string)
                n154 = Concatenate Strings(w345, w346) -> (w347:string)
              }
              n155 = call "Write_File_Simple.vi"("append to file? (new file:F)"=FALSE, "character string"=w335, "file path"=w333) -> ()  [unwired: 2 out]
            }
            frame 1 {
              n156 = local read "# total vectors"() -> (w352:i32)
              n157 = Number To Decimal String(number=w352) -> (decimal integer string=w351:string)  [unwired: 1 in]
              n158 = Build Array (concatenate)(string[] ["EnSight Model Geometry File", "EnSight 9.2 ", "node id assign", "element id assign", "part", "         1", "Point field", "coordinates"], w351) -> (w350:string[])
              n159 = for {
                tunnel: w350 -> [w362] mode=indexing
                shift-right: [w360] -> w356
                shift-left: "" -> [w358]
                n160 = Concatenate Strings(w362, "\n") -> (w359:string)
                n161 = Concatenate Strings(w358, w359) -> (w360:string)
              }
              n162 = call "Write_File_Simple.vi"("append to file? (new file:F)"=FALSE, "character string"=w356, "file path"=w354) -> ()  [unwired: 2 out]
            }
            frame 2, Default {
              n163 = local read "Variable Names"() -> (w369:string[])
              n164 = Subtract(x=w368, y=2) -> (x-y=w366:i32)
              n165 = Index Array(array=w369, index=w366) -> (element=w365:string)
              n166 = Build Array (concatenate)(w365, string[] ["part", "         1", "coordinates"]) -> (w363:string[])
              n167 = for {
                tunnel: w363 -> [w378] mode=indexing
                shift-right: [w376] -> w371
                shift-left: "" -> [w374]
                n168 = Concatenate Strings(w378, "\n") -> (w375:string)
                n169 = Concatenate Strings(w374, w375) -> (w376:string)
              }
              n170 = call "Write_File_Simple.vi"("append to file? (new file:F)"=FALSE, "character string"=w371, "file path"=w373) -> ()  [unwired: 2 out]
            }
          }
        }
      }
      frame "Collect Data" {
        w383 = T2 []  # Array
        n171 = for {
          N -> [w394]
          tunnel: w385 -> [w402] mode=indexing
          tunnel: [w400] -> w379 mode=indexing
          tunnel: [w399] -> w381 mode=indexing
          i -> [w395]
          n172 = Unbundle By Name(w402) -> ("Record Length"=w401:dbl, "Turb Stats"=w393:T4, "Turb Stats Error"=w390:T4, "XYZ Position"=w399:dbl[])
          n173 = Divide(x=w395, y=w394) -> (x/y=w397:dbl)
          n174 = Multiply(x=w397, y=100) -> (x*y=w398:dbl)
          n175 = local write "Progress Bar"(w398) -> ()
          n176 = Index Array(array=w393) -> (element=w392:T3)  [unwired: 1 in]
          n177 = Index Array(array=w390) -> (element=w389:T3)  [unwired: 1 in]
          n178 = Cluster To Array(cluster=w392) -> (array=w391:dbl[])
          n179 = Cluster To Array(cluster=w389) -> (array=w388:dbl[])
          n180 = Build Array (concatenate)(w401, w391, w388) -> (w400:dbl[])
        }
        "Data Array (spot,Var)" <- w379
        n181 = local write "Status"("Gathering all the data ready to write to file..." ("Status")) -> ()
        n182 = Transpose 2D Array(2D array=w381) -> (transposed array=→"Position Array (XYZ,spot)":dbl[][])
      }
      frame "Save Data" {
        n183 = local read "Data Array (spot,Var)"() -> (w407:dbl[][])
        n184 = local read "Position Array (XYZ,spot)"() -> (w406:dbl[][])
        n185 = local read "File Paths"() -> (w408:path[])
        n186 = Transpose 2D Array(2D array=w407) -> (transposed array=w403:dbl[][])
        n187 = local write "Status"("Wrting the data to file..." ("Status")) -> ()
        n188 = for {
          N -> [w412]
          tunnel: w408 -> [w419] mode=indexing
          tunnel: w403 -> [w418]
          tunnel: w406 -> [w417]
          i -> [w413]
          # "Loop Variable"
          n189 = Divide(x=w413, y=w412) -> (x/y=w415:dbl)
          n190 = Multiply(x=w415, y=100) -> (x*y=w416:dbl)
          n191 = local write "Progress Bar"(w416) -> ()
          n192 = case shown="2, Default" w413 {
            tunnel: w419 -> [_ w425 w437]
            tunnel: w413 -> [_ _ w444]
            tunnel: w418 -> [_ _ w441]
            tunnel: w417 -> [_ w424 _]
            frame 0 {
            }
            frame 1 {
              n193 = Index Array(array=w424) -> (element #1=w423:dbl[], element #2=w422:dbl[], element #3=w421:dbl[])  [unwired: 6 in]
              n194 = Build Array (concatenate)(w423, w422, w421) -> (w420:dbl[])
              n195 = for {
                tunnel: w420 -> [w429] mode=indexing
                shift-right: [w435] -> w426
                shift-left: "" -> [w434]
                w430 = T5 4 items=["no dialog", "OK message", "continue or stop message", "OK message + warnings", "continue/stop + warnings"] ("type of dialog (OK msg:1)")
                n196 = call "Ensight_Format_Check.vi"("Input Number"=w429) -> ("error"=w432:errorcluster, "Output string"=w433:string)  [unwired: 8 in, 1 out]
                n197 = Concatenate Strings(w434, w433) -> (w435:string)
                n198 = call <vilib>:"Simple Error Handler.vi"("error source (\" \")"="GEOM" ("error source (\" \")"), "type of dialog (OK msg:1)"=w430, "error in (no error)"=w432) -> ()  [unwired: 2 in, 5 out]
              }
              n199 = call "Write_File_Simple.vi"("append to file? (new file:F)"=TRUE, "character string"=w426, "file path"=w425) -> ()  [unwired: 2 out]
            }
            frame 2, Default {
              n200 = Subtract(x=w444, y=2) -> (x-y=w436:i32)
              n201 = Index Array(array=w441, index (row)=w436) -> (element=w440:dbl[])  [unwired: 1 in]
              n202 = for {
                tunnel: w440 -> [w445] mode=indexing
                shift-right: [w454] -> w438
                shift-left: "" -> [w453]
                tunnel: w437 -> [w450]
                w446 = T5 4 items=["no dialog", "OK message", "continue or stop message", "OK message + warnings", "continue/stop + warnings"] ("type of dialog (OK msg:1)")
                n203 = Path To String(path=w450) -> (string=w449:string)
                n204 = call "Ensight_Format_Check.vi"("Input Number"=w445) -> ("error"=w451:errorcluster, "Output string"=w452:string)  [unwired: 8 in, 1 out]
                n205 = Concatenate Strings("VAR file: " ("error source (\" \")"), w449) -> (w447:string)
                n206 = call <vilib>:"Simple Error Handler.vi"("error source (\" \")"=w447, "type of dialog (OK msg:1)"=w446, "error in (no error)"=w451) -> ()  [unwired: 2 in, 5 out]
                n207 = Concatenate Strings(w453, w452) -> (w454:string)
              }
              n208 = call "Write_File_Simple.vi"("append to file? (new file:F)"=TRUE, "character string"=w438, "file path"=w437) -> ()  [unwired: 2 out]
            }
          }
        }
      }
      frame "End Time" {
        n209 = local write "Position Array (XYZ,spot)"(dbl[][] [] ("Position Array")) -> ()
        n210 = local write "Data Array (spot,Var)"(dbl[][] [] ("Data Array")) -> ()
      }
    }
  }
  "Progress Bar" <- u8 0 ("Progress Bar")
